vi "TreePriorityColoring.vi"(7 "Color Array":u32[](array[colorbox]), 8 "Error In":errorcluster, 10 "Tree Refnum":refnum<vi>, 11 "SR List In":T1[](array[typedef])) -> (0 "Error Out":errorcluster, 3 "SR Count per Prio":u32[](array[numeric]))   [LabVIEW 2017, in "Client.lvlib" / "UI_API.lvlib"]
uses:
  UI_API.lvlib
  ParserSorter/TypeDefs/SRData.ctl
  ParserSorter/TypeDefs/AEGroup.ctl
  ParserSorter/TypeDefs/SRStatus.ctl
  ParserSorter/TypeDefs/SRLevel.ctl
  ParserSorter/TypeDefs/SRType.ctl
  8f031662-b8fd-4488-80a1-5f4451c664a6.vi
  8a47623c-d043-40bb-a838-40019f94e353.vi
  f1c03f4c-73db-46dc-83ec-66573ffbbd34.vi
  4dfd4452-9ebc-4416-8a52-64a9d7b80120.vi
  ParserSorter/ParserSorter.lvlib
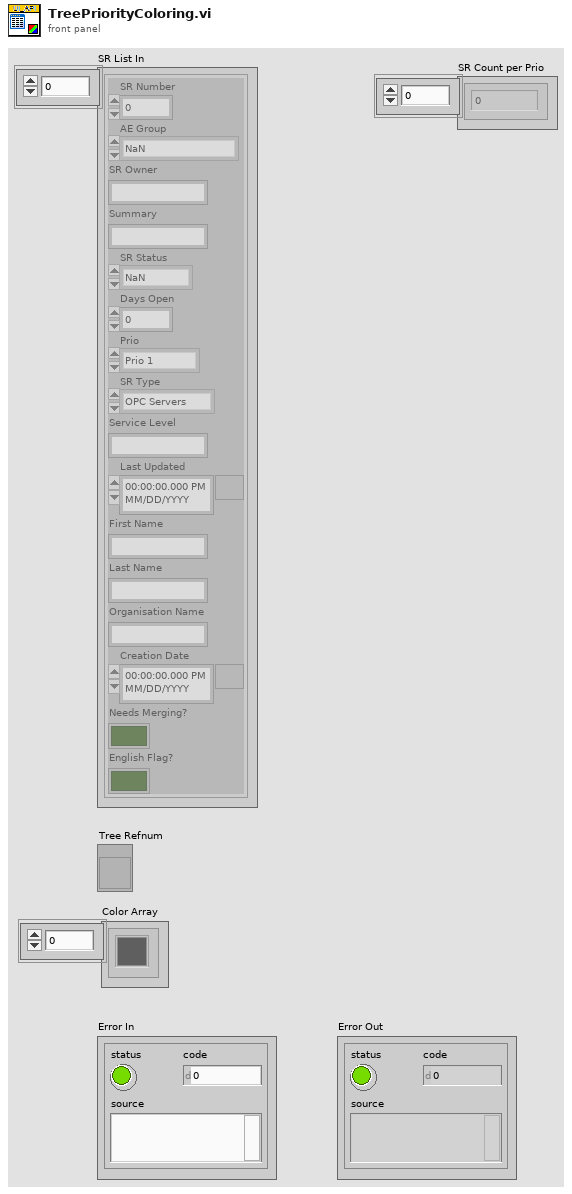
[diagram p1: front panel]
types:
  T1 = typedef "Client.lvlib/ParserSorter.lvlib/SRData.ctl" = cluster{"SR Number":i64, "AE Group":T2, "SR Owner":string, "Summary":string, "SR Status":T3, "Days Open":dbl, "Prio":T4, "SR Type":T5, "Service Level":string, "Last Updated":timestamp, "First Name":string, "Last Name":string, "Organisation Name":string, "Creation Date":timestamp, "Needs Merging?":bool, "English Flag?":bool}
  T2 = typedef "Client.lvlib/ParserSorter.lvlib/AEGroup.ctl" = enum32{"NaN", "AE-Germany", "AE-Poland", "AE-Switzerland", "AE-Czech Republic", "AE-Hungary", "AE-Romania", "AE-Slovakia", "AE-Slovenia"}
  T3 = typedef "Client.lvlib/ParserSorter.lvlib/SRStatus.ctl" = enum32{"NaN", "Caller Abandoned", "Created in Error", "Declined to Purchase Support", "Expired", "Forum Resolved AE", "Forum Resolved Customer", "IN WORK", "IN WORK Collab with AES", "IN WORK Collab with PSE", "IN WORK Collab with SE", "IN WORK Escalation", "IN WORK Customer Added Note", "Open", "Potentially Resolved", "POC Resolved", "Resolved", "RMA Waiting on Customer", "RMA Open", "RMA In Progress", "RMA Closed - DOA", "RMA Closed", "RMA Approved for Return", "Project Complete", "Presumed Resolved", "IN WORK Wait on Customer"}
  T4 = typedef "Client.lvlib/ParserSorter.lvlib/SRLevel.ctl" = enum16{"Prio 1", "Prio 2", "Prio 3", "Prio 4"}
  T5 = typedef "Client.lvlib/ParserSorter.lvlib/SRType.ctl" = enum32{"NaN", "ATE Core Configurations (BYOATE)", "Activation", "BioBench", "CAN", "CM C Series", "Calibration", "Consulting Services", "CounterTimer", "DAQExpress", "DASYLab", "DIAdem", "DMM", "DSA HW", "Digital_IO", "FIRST (NIC Only)", "FieldBus", "FieldPoint", "Functional Savety", "GATI", "GPIB", "HMI and Industrial PCs", "HiQ", "HighSpeedDigital_IO", "IMAQ", "IOTech Vibration", "Industrial Communications", "InsightCM", "LV", "LV CD&Sim", "LV Comms", "LV Controls Add-Ons", "LV Embedded", "LV MathScript RT", "LV NXG", "LV NXT", "LVDSC", "LVFPGA", "LVPDA and LV Touch Panel", "LVRT", "LabWindows_CVI", "Lookout", "MATRIXx", "MStudioDotNet", "MStudioVisualBasic", "MStudioVisualC", "Measure (Legacy)", "Motion", "MultifunctionDAQ", "Multimedia Test HW/SW", "Multisim (EWB)", "NI Update Service", "OPC Servers", "Optical (OSI)", "PXI Controllers, Chassis, MXI", "PXI Timing and Sync", "Power Supplies and SMUs", "Powertrain Controls", "RAID", "RF", "RF Software", "RIO", "SC Express", "SCC", "SCXI", "SPEEDY-33 (Hyperception)", "STS", "ScopeDigitizers", "Serial", "Signal Sources", "SignalCondOther", "SignalExpress", "Software Defined Intruments", "Sound and Vibration SW", "Switch Executive", "Switches", "TestStand", "USRP", "Ultiboard (EWB)", "VBench", "VI Logger", "VXI_MXI", "VeriStand", "VisionSW", "VolumeLicenseMgr", "WSN", "Web UI Builder", "myRIO"}
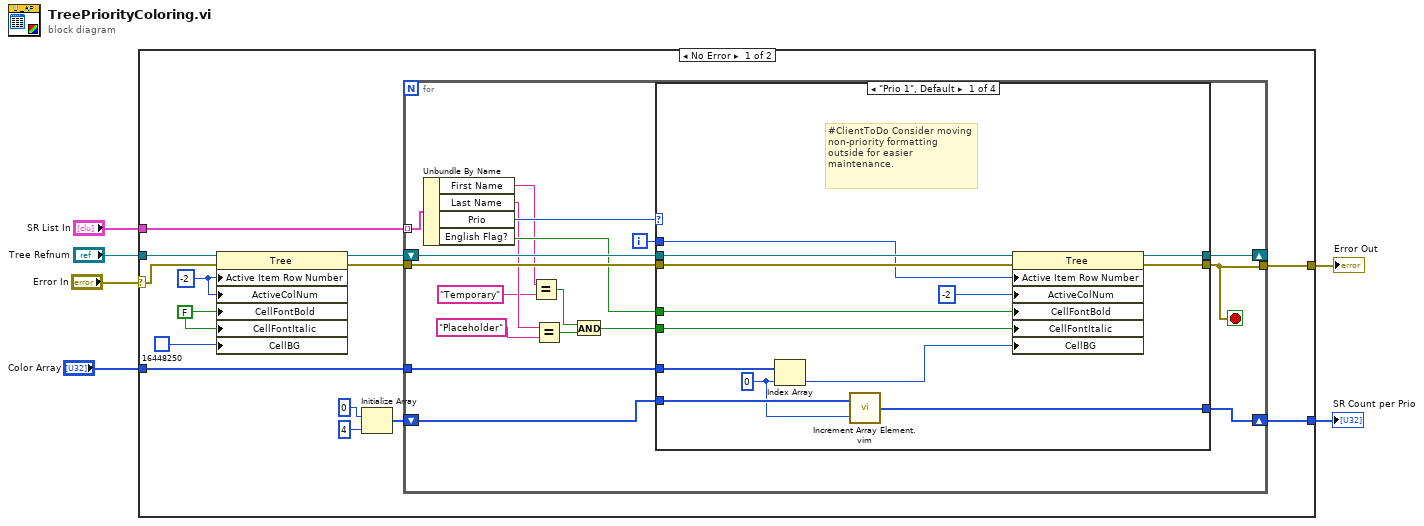
[diagram p0: block diagram]
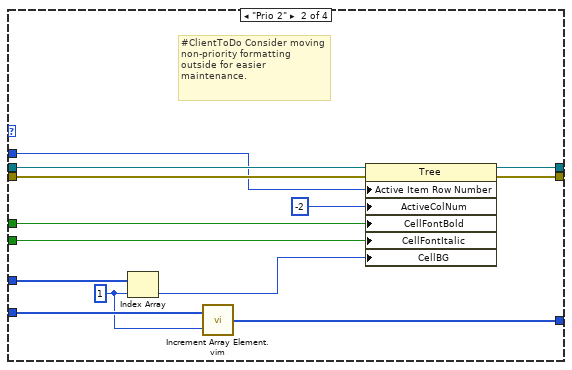
[diagram p2: hidden frame]
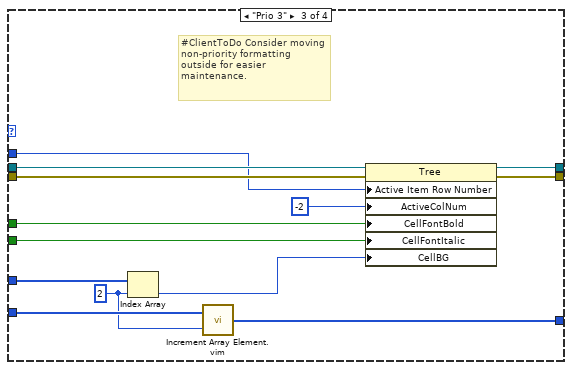
[diagram p3: hidden frame]
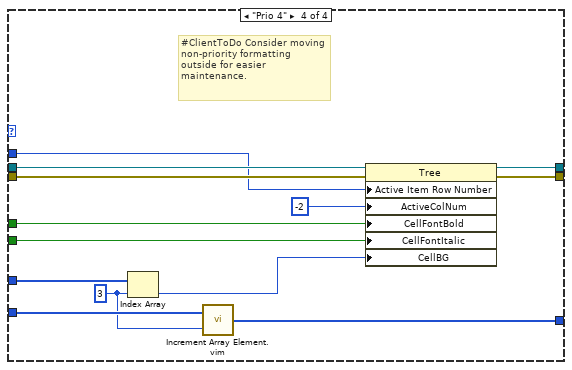
[diagram p4: hidden frame]
diagram:
  n1 = case shown="No Error" "Error In" {
    selector: "Error In" -> [w12 w91]
    tunnel: "SR List In" -> [w20 _]
    tunnel: "Tree Refnum" -> [w13 _]
    tunnel: "Color Array" -> [w18 _]
    tunnel: [w19 w91] -> w2
    tunnel: [w14 _] -> w1
    frame No Error {
      w7 = -2 ("Column")
      w11 = FALSE ("Active Cell:Cell Font:Italic")
      n2 = property on="Property Node" class="Tree"(reference=w13, error in=w12, "Active Item Row Number"=w7, "ActiveColNum"=w7, "CellFontBold"=w11, "CellFontItalic"=w11, "CellBG"=u32 16448250) -> (reference out=w9:refnum<vi>, error out=w8:errorcluster)
      n3 = Initialize Array(u32 0, 4 ("dimension size")) -> (w15:u32[])
      n4 = for {
        tunnel: w20 -> [w38] mode=indexing
        tunnel: w18 -> [w36]
        shift-right: [w34] -> _
        shift-left: w9 -> [w37]
        tunnel: w8 -> [w33]
        tunnel: [w32] -> w19
        shift-right: [w21] -> w14
        shift-left: w15 -> [w22]
        i -> [w35]
        stop <- w32 stop-if-true
        n5 = Unbundle By Name(w38) -> ("First Name"=w26:string, "Last Name"=w25:string, "Prio"=w31:T4, "English Flag?"=w30:bool)
        n6 = Equal?(x=w26, y="Temporary") -> (x = y?=w29:bool)
        n7 = Equal?(x=w25, y="Placeholder") -> (x = y?=w28:bool)
        n8 = And(x=w29, y=w28) -> (x .and. y?=w27:bool)
        n9 = case shown="\"Prio 1\", Default" w31 {
          tunnel: w37 -> [w46 w59 w72 w85]
          tunnel: w36 -> [w51 w64 w77 w90]
          tunnel: w35 -> [w44 w57 w70 w83]
          tunnel: [w48 w61 w74 w87] -> w34
          tunnel: w33 -> [w45 w58 w71 w84]
          tunnel: [w47 w60 w73 w86] -> w32
          tunnel: w30 -> [w41 w54 w67 w80]
          tunnel: w27 -> [w40 w53 w66 w79]
          tunnel: w22 -> [w50 w63 w76 w89]
          tunnel: [w49 w62 w75 w88] -> w21
          frame "Prio 1", Default {
            w39 = 0 ("index")
            # "#ClientToDo Consider moving non-priority formatting outside for easier maintenance."
            n10 = Index Array(array=w51, index=w39) -> (element=w42:u32)
            n11 = call "Increment Array Element.vim"("index"=w39, "array in"=w50) -> ("array out"=w49:u32[])
            n12 = property on="Property Node" class="Tree"(reference=w46, error in=w45, "Active Item Row Number"=w44, "ActiveColNum"=-2 ("Column"), "CellFontBold"=w41, "CellFontItalic"=w40, "CellBG"=w42) -> (reference out=w48:refnum<vi>, error out=w47:errorcluster)
          }
          frame "Prio 2" {
            w52 = 1 ("index")
            # "#ClientToDo Consider moving non-priority formatting outside for easier maintenance."
            n13 = Index Array(array=w64, index=w52) -> (element=w55:u32)
            n14 = call "Increment Array Element.vim"("index"=w52, "array in"=w63) -> ("array out"=w62:u32[])
            n15 = property on="Property Node" class="Tree"(reference=w59, error in=w58, "Active Item Row Number"=w57, "ActiveColNum"=-2 ("Column"), "CellFontBold"=w54, "CellFontItalic"=w53, "CellBG"=w55) -> (reference out=w61:refnum<vi>, error out=w60:errorcluster)
          }
          frame "Prio 3" {
            w65 = 2 ("index")
            # "#ClientToDo Consider moving non-priority formatting outside for easier maintenance."
            n16 = Index Array(array=w77, index=w65) -> (element=w68:u32)
            n17 = call "Increment Array Element.vim"("index"=w65, "array in"=w76) -> ("array out"=w75:u32[])
            n18 = property on="Property Node" class="Tree"(reference=w72, error in=w71, "Active Item Row Number"=w70, "ActiveColNum"=-2 ("Column"), "CellFontBold"=w67, "CellFontItalic"=w66, "CellBG"=w68) -> (reference out=w74:refnum<vi>, error out=w73:errorcluster)
          }
          frame "Prio 4" {
            w78 = 3 ("index")
            # "#ClientToDo Consider moving non-priority formatting outside for easier maintenance."
            n19 = Index Array(array=w90, index=w78) -> (element=w81:u32)
            n20 = call "Increment Array Element.vim"("index"=w78, "array in"=w89) -> ("array out"=w88:u32[])
            n21 = property on="Property Node" class="Tree"(reference=w85, error in=w84, "Active Item Row Number"=w83, "ActiveColNum"=-2 ("Column"), "CellFontBold"=w80, "CellFontItalic"=w79, "CellBG"=w81) -> (reference out=w87:refnum<vi>, error out=w86:errorcluster)
          }
        }
      }
    }
    frame Error {
    }
  }
  "Error Out" <- w2
  "SR Count per Prio" <- w1
